vi "ClientSrv Client.vi"() -> ()   [LabVIEW 2012]
doc: "This client VI can connect to a remote server and provides a start menu to open the various user interface windows needed to control and monitor that server. To avoid confusion, no simultaneous connections to multiple servers are allowed. This client and the user interfaces it manages are designed to access a remote server over a TCP/IP network, but are also able to connect to a server running in the same LabVIEW runtime environment. A local connection is convenient for testing during development, and leaves open the option of building a single executable that includes both the client and server. The latter is not advisable since the segregation of the client-side user interfaces from the server not only provides for remote access, but also offloads work and complexity from the server, thereby improving its performance and robustness.\n\nVia the \"server\" menu, a server can be connected to. When a connection to an as yet unkown server is succesfully established, a preset is added that allows a quick reconnection without the need for respecifying the machine name and port number. When disconnecting, the server session is stored. The \"session\" is comprised of the positions, sizes, open/closed state, as well as the persistent controls of the user interface windows. When reconnecting, the previous session is restored.\n\nThe runlevels of the server to which a connection has been established are displayed in a submenu. The attained runlevel is indicated with a checkmark. Using this submenu it is possible to switch the server between runlevels. This operation requires operator access. Note that the runlevels menu does not update while it or some other menu is held open."
uses:
  served/ClientSrv Server Runlevels_srv.ctl
  luaview/served/LuaVIEW Info_srv.ctl
  typedefs/t_ClientSrv Client Main States.ctl
  typedefs/t_ClientSrv Server Runlevels Methods.ctl
  typedefs/t_ClientSrv Access Levels.ctl
  typedefs/t_ClientSrv Client Access State Methods.ctl
  library/typedefs/t_Library Session Methods.ctl
  luaview/typedefs/clusters/LuaVIEW Task Console Ancillary.ctl
  typedefs/t_ClientSrv Connection State Methods.ctl
  subvis/private/glb_ClientSrv Globals.vi
  <vilib>/Platform/browser.llb/Open URL in Default Browser (string).vi
panel:
  in  "local path":path
  in  "editor command":string="notepad \"<file>\""
  out "rebootmode":string
  out "info":T1
  out "runlevels":T2
  out "server":string
  out "remember":bool
  out "observer digest":string
  out "port number":u32
  out "machine name":string
  in  "presets":T3(array[cluster])
  in  "list":i32(listbox)
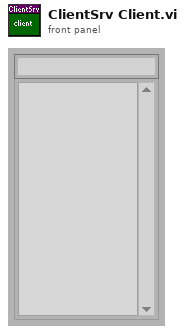
[diagram p1: front panel]
types:
  T1 = typedef "LuaVIEW Info_srv.ctl" = refnum<vi>
  T2 = typedef "ClientSrv Server Runlevels_srv.ctl" = refnum<vi>
  T3 = cluster{"server":string, "machine":string, "port":u32, "digest":string, "remember":bool}[]
  T4 = typedef "t_ClientSrv Client Main States.ctl" = enum16{"empty queue", "poll list selection", "browse editor", "set editor", "no editors?", "<3 editors?", "remote file", "connect", "stop session", "server stop", "server reboot", "disconnect", "open refs", "update presets", "update name", "update ablement", "update sizes", "start session", "run consoles", "initialize", "init title", "init disconnect", "init patience", "init persist", "init paths", "init list", "init sort", "init done", "cleanup", "stop"}
  T5 = typedef "t_ClientSrv Server Runlevels Methods.ctl" = enum16{"get levels", "get modes", "change", "set bootmode"}
  T6 = typedef "t_ClientSrv Access Levels.ctl" = enum16{"observer", "operator", "local"}
  T7 = typedef "t_ClientSrv Client Access State Methods.ctl" = enum16{"ensure", "release"}
  T8 = typedef "LuaVIEW Task Console Ancillary.ctl" = cluster{"open on start":bool, "stop on close":bool, "hide initial":bool, "timeout":u32}
  T9 = typedef "t_Library Session Methods.ctl" = enum16{"run", "get arg", "set arg", "delist", "cleanup?", "start session", "stop session", "list empty?"}
  T10 = typedef "t_ClientSrv Connection State Methods.ctl" = enum16{"connect", "get state", "disconnect"}
  T11 = enum32{"invalid app kind", "Development System", "Run Time System", "Student Edition", "Embedded LabVIEW", "Evaluation", "Custom"}
  T12 = enum32{"existing file", "new file", "new or existing file", "existing dir", "new dir", "new or existing dir", "existing file (use LLBs)", "new file (use LLBs)", "new or existing file (use LLBs)", "new or existing file or directory (use LLBs)"}
  T13 = cluster{"server":string, "machine":string, "port":u32, "digest":string, "remember":bool}
  T14 = typedef "eventvkey.ctl" = enum16{"ASCII", "Enter", "Return", "Shift", "Ctrl", "Alt", "Cmd", "Opt", "Caps", "NumLock", "Clear", "Break", "Up", "Down", "Left", "Right", "Insert", "Delete", "Home", "End", "PageUp", "PageDown", "Escape", "Help", "Pause", "ScrollLock", "F1", "F2", "F3", "F4", "F5", "F6", "F7", "F8", "F9", "F10", "F11", "F12", "F13", "F14", "F15", "F16", "F17", "F18", "F19", "F20", "F21", "F22", "F23", "F24", "Play", "VolumeUp", "VolumeDown", "Mute", "Two Byte Char"}
  T15 = enum32{"Bad", "Idle", "Run top level", "Running"}
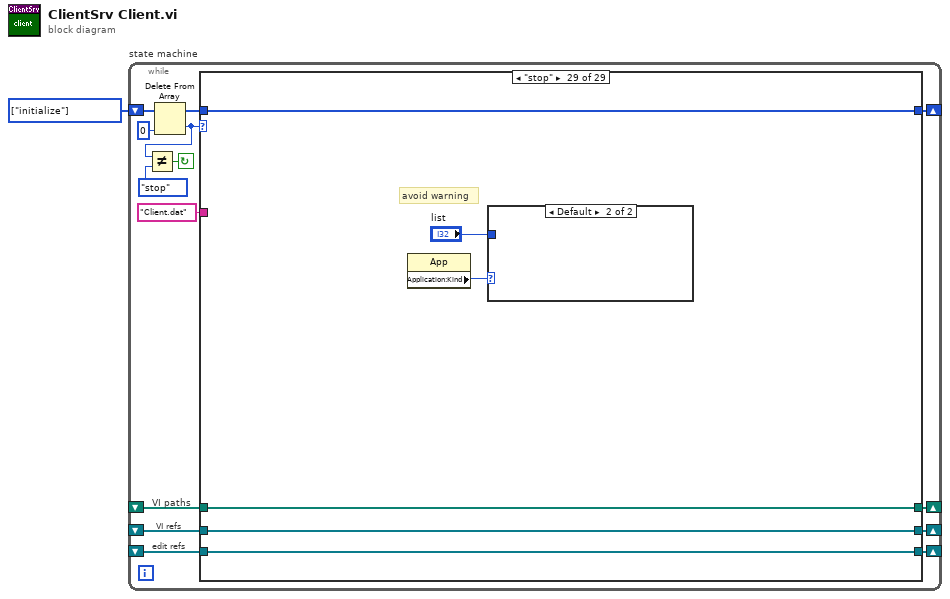
[diagram p0: block diagram]
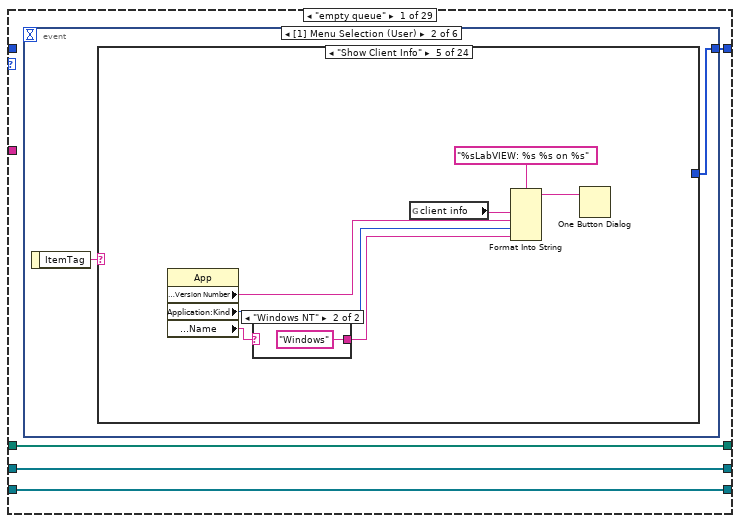
[diagram p2: hidden frame]
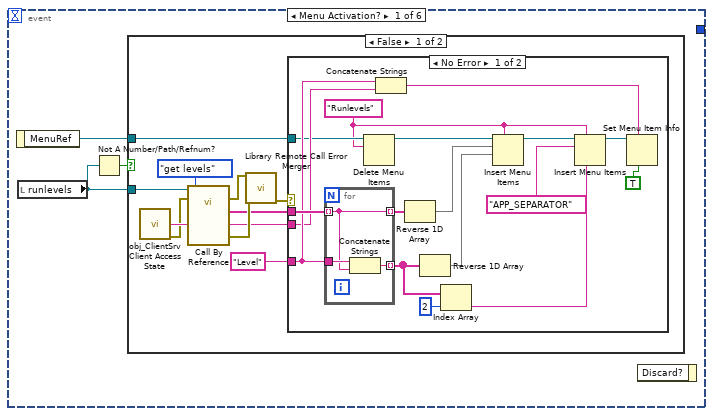
[diagram p3: hidden frame]
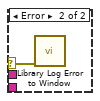
[diagram p4: hidden frame]
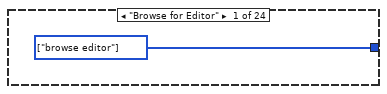
[diagram p6: hidden frame]
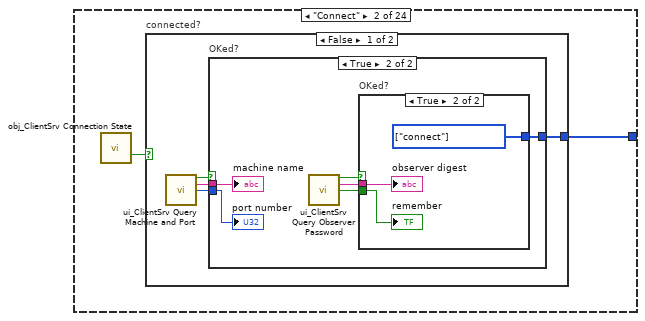
[diagram p7: hidden frame]
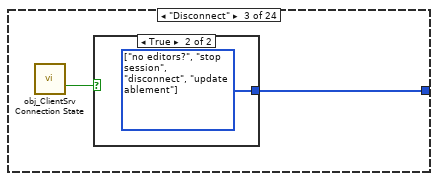
[diagram p11: hidden frame]
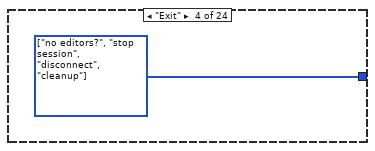
[diagram p13: hidden frame]
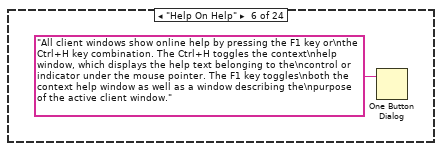
[diagram p15: hidden frame]
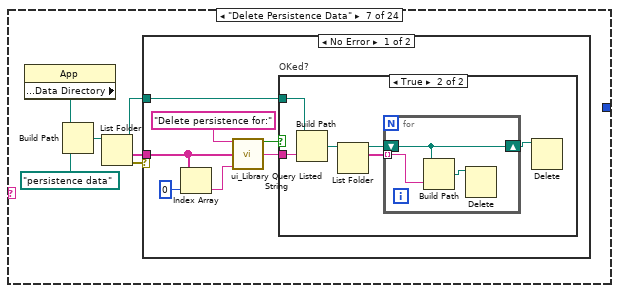
[diagram p16: hidden frame]
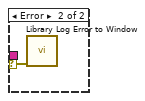
[diagram p18: hidden frame]
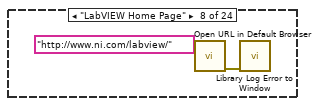
[diagram p19: hidden frame]
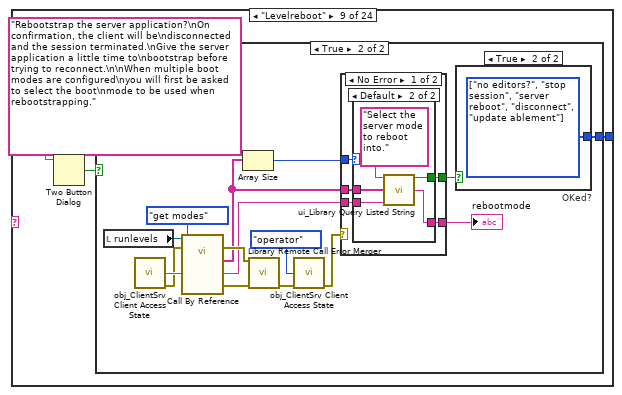
[diagram p20: hidden frame]
diagram:
  w1 = T4[] [enum."initialize"] items=["empty queue", "poll list selection", "browse editor", "set editor", "no editors?", "<3 editors?", "remote file", "connect", "stop session", "server stop", "server reboot", "disconnect", "open refs", "update presets", "update name", "update ablement", "update sizes", "start session", "run consoles", "initialize", "init title", "init disconnect", "init patience", "init persist", "init paths", "init list", "init sort", "init done", "cleanup", "stop"] ("Array Constant")
  n1 = while "state machine" {
    shift-left: w1 -> [w13]
    shift-right: [w15] -> _
    shift-right: [w9] -> _
    shift-left: _ -> [w10]
    shift-right: [w7] -> _
    shift-left: _ -> [w8]
    shift-right: [w3] -> _
    shift-left: _ -> [w2]
    stop <- w14 continue-if-true
    # "edit refs"
    # "VI paths"
    # "VI refs"
    n2 = Delete From Array(array=w13, index=0) -> (deleted portion=w5:T4, array with subset deleted=w12:T4[])  [unwired: 1 in]
    n3 = Not Equal?(x=w5, y=t_ClientSrv_Client_Main_States."stop" ("states")) -> (x != y?=w14:bool)
    n4 = case "Case" shown="\"stop\"" w5 {
      selector: w5 -> [_ _ w318 _ _ _ _ _ _ _ _ _ _ _ _ _ _ _ _ _ _ _ _ _ _ _ _ _ _]
      tunnel: [w19 w309 w322 w345 w369 w408 w424 w430 w455 w460 w479 w508 w570 w604 w647 w668 w673 w689 w693 w722 w727 w736 w740 w753 w771 w852 w865 w882 w892] -> w15
      tunnel: w12 -> [_ w309 w322 w346 w370 w408 _ w430 w455 w460 w479 w508 w570 w604 w647 w668 w673 w689 _ w722 w727 w736 w741 w752 w770 w852 w866 _ w892]
      tunnel: w10 -> [w18 w305 w321 w352 w379 w410 w425 w432 w457 w476 w481 w507 w571 w605 w648 w669 w674 w688 w692 w724 w729 w737 w745 w749 _ w846 w867 w876 w890]
      tunnel: [w18 w305 w321 w352 w379 w410 w425 w432 w457 w476 w481 w507 w571 w605 w648 w669 w674 w688 w692 w724 w729 w737 w745 w749 w766 w846 w867 w875 w890] -> w9
      tunnel: w8 -> [w17 w307 w320 w351 w378 w409 w423 w431 w456 w475 w480 w506 w568 w603 w646 w667 w672 w687 w691 w723 w728 w735 w743 _ w767 w848 w863 w877 w889]
      tunnel: [w17 w306 w320 w351 w378 w409 w423 w431 w456 w475 w480 w506 w568 w603 w646 w667 w672 w687 w691 w723 w728 w735 w743 w750 w767 w847 w863 w878 w889] -> w7
      tunnel: "Client.dat" ("filename (<window title>.dat)") -> [_ _ _ _ _ _ _ _ _ _ _ _ _ _ _ _ _ _ _ _ _ _ w742 _ _ _ _ w871 _]
      tunnel: [w16 w299 w316 w347 w374 w397 w417 w429 w445 w458 w477 w501 w551 w592 w618 w660 w670 w675 w690 w719 w725 w730 w738 w747 w765 w843 w861 w868 w887] -> w3
      tunnel: w2 -> [w16 w299 w316 w350 w377 w396 w417 w429 w445 w458 w477 w501 w551 w592 w618 w660 w670 w675 w690 w719 w725 w730 w738 w747 w765 w843 w861 w868 w887]
      frame "empty queue" {
        n5 = event shown="[1] Menu Selection (User)" {
          selector: _ -> [_ _ _ _ _ _]
          dyn-events: _ -> [_ _ _ _ _ _]
          timeout: _ -> [_ _ _ _ _ _]
          tunnel: [_ w56 w286 _ w297 w298] -> w19
          event Menu Activation? {
            n6 = event-data() -> ("MenuRef"=w20:refnum<k9>)  [unwired: 1 in]
            n7 = local read "runlevels"() -> (w21:T2)
            n8 = Not A Number/Path/Refnum?(number/path/refnum=w21) -> (NaN/Path/Refnum?=w22:bool)
            n9 = case shown="False" w22 {
              tunnel: w21 -> [w33 _]
              tunnel: w20 -> [w23 _]
              frame False {
                n10 = call "obj_ClientSrv Client Access State.vi"() -> ("certificate"=w31:string, "error out"=w30:errorcluster)  [unwired: 14 in]
                n11 = call-by-ref "?"(reference=w33, error in=w30, "method"=t_ClientSrv_Server_Runlevels_Methods."get levels", "certificate"=w31) -> (error out=w29:errorcluster, "names"=w26:string[], "current"=w25:string, 15:"error out"=w28:errorcluster)  [unwired: 11 in, 1 out]
                n12 = call "Library Remote Call Error Merger.vi"("call by reference node error"=w29, "called VI error (no error)"=w28) -> ("error out"=w27:errorcluster)  [unwired: 13 in]
                n13 = case shown="No Error" w27 {
                  selector: w27 -> [_ w54]
                  tunnel: w26 -> [w49 _]
                  tunnel: w25 -> [w47 _]
                  tunnel: "Level" ("menu tag") -> [w48 _]
                  tunnel: w23 -> [w43 _]
                  frame No Error {
                    w41 = "Runlevels" ("menu tag")
                    n14 = for {
                      tunnel: w49 -> [w52] mode=indexing
                      tunnel: [w52] -> w46 mode=indexing
                      tunnel: w48 -> [w53]
                      tunnel: [w51] -> w36 mode=indexing
                      n15 = Concatenate Strings(w53, w52) -> (w51:string)
                    }
                    n16 = Delete Menu Items(8:w41, 9:w43) -> (3:w50:refnum<k9>)  [unwired: 2 in, 1 out]
                    n17 = Concatenate Strings(w48, w47) -> (w45:string)
                    n18 = Reverse 1D Array(array=w46) -> (reversed array=w37:string[])
                    n19 = Reverse 1D Array(array=w36) -> (reversed array=w38:string[])
                    n20 = Index Array(array=w36, index=2) -> (element=w34:string)
                    n21 = Insert Menu Items(5:w41, 7:w38, 8:w37, 9:w50) -> (3:w40:refnum<k9>)  [unwired: 2 in, 2 out]
                    n22 = Insert Menu Items(4:w34, 5:w41, 8:"APP_SEPARATOR" ("after item"), 9:w40) -> (3:w42:refnum<k9>)  [unwired: 2 in, 2 out]
                    n23 = Set Menu Item Info(6:TRUE ("checked"), 7:w45, 11:w42) -> ()  [unwired: 4 in, 2 out]
                  }
                  frame Error {
                    n24 = call "Library Log Error to Window.vi"("error in (no error)"=w54) -> ()  [unwired: 13 in, 2 out]
                  }
                }
              }
              frame True {
              }
            }
            n25 = event-data() -> ()  [unwired: 2 in, 1 out]
          }
          event Menu Selection (User) {
            n26 = event-data() -> ("ItemTag"=w55:string)  [unwired: 1 in]
            n27 = case shown="\"Show Client Info\"" w55 {
              selector: w55 -> [_ _ _ _ _ _ _ _ _ _ _ _ _ _ _ _ _ _ _ _ _ _ _ w201]
              tunnel: [w57 w59 w74 w76 _ _ _ _ w112 w143 _ _ _ _ _ _ _ w174 w175 _ _ _ _ w202] -> w56
              frame "Browse for Editor" {
                w57 = T4[] [enum."browse editor"] items=["empty queue", "poll list selection", "browse editor", "set editor", "no editors?", "<3 editors?", "remote file", "connect", "stop session", "server stop", "server reboot", "disconnect", "open refs", "update presets", "update name", "update ablement", "update sizes", "start session", "run consoles", "initialize", "init title", "init disconnect", "init patience", "init persist", "init paths", "init list", "init sort", "init done", "cleanup", "stop"] ("Array Constant")
              }
              frame "Connect" {
                n28 = call "obj_ClientSrv Connection State.vi"() -> ("connected?"=w58:bool)  [unwired: 8 in, 7 out]
                n29 = case "connected?" shown="False" w58 {
                  tunnel: [w60 _] -> w59
                  frame False {
                    n30 = call "ui_ClientSrv Query Machine and Port.vi"() -> ("OKed?"=w63:bool, "machine name out"=w62:string, "port number out"=w61:u32)  [unwired: 13 in]
                    n31 = case "OKed?" shown="True" w63 {
                      tunnel: w62 -> [_ w68]
                      tunnel: w61 -> [_ w67]
                      tunnel: [_ w69] -> w60
                      frame False {
                      }
                      frame True {
                        n32 = call "ui_ClientSrv Query Observer Password.vi"() -> ("OKed?"=w66:bool, "observer digest"=w65:string, "remember out"=w64:bool)  [unwired: 13 in]
                        n33 = case "OKed?" shown="True" w66 {
                          tunnel: [_ w70] -> w69
                          tunnel: w65 -> [_ w72]
                          tunnel: w64 -> [_ w71]
                          frame False {
                          }
                          frame True {
                            w70 = T4[] [enum."connect"] items=["empty queue", "poll list selection", "browse editor", "set editor", "no editors?", "<3 editors?", "remote file", "connect", "stop session", "server stop", "server reboot", "disconnect", "open refs", "update presets", "update name", "update ablement", "update sizes", "start session", "run consoles", "initialize", "init title", "init disconnect", "init patience", "init persist", "init paths", "init list", "init sort", "init done", "cleanup", "stop"] ("Array Constant")
                            "observer digest" <- w72
                            "remember" <- w71
                          }
                        }
                        "machine name" <- w68
                        "port number" <- w67
                      }
                    }
                  }
                  frame True {
                  }
                }
              }
              frame "Disconnect" {
                n34 = call "obj_ClientSrv Connection State.vi"() -> ("connected?"=w73:bool)  [unwired: 8 in, 7 out]
                n35 = case shown="True" w73 {
                  tunnel: [_ w75] -> w74
                  frame False {
                  }
                  frame True {
                    w75 = T4[] [enum."no editors?", enum."stop session", enum."disconnect", enum."update ablement"] items=["empty queue", "poll list selection", "browse editor", "set editor", "no editors?", "<3 editors?", "remote file", "connect", "stop session", "server stop", "server reboot", "disconnect", "open refs", "update presets", "update name", "update ablement", "update sizes", "start session", "run consoles", "initialize", "init title", "init disconnect", "init patience", "init persist", "init paths", "init list", "init sort", "init done", "cleanup", "stop"] ("Array Constant")
                  }
                }
              }
              frame "Exit" {
                w76 = T4[] [enum."no editors?", enum."stop session", enum."disconnect", enum."cleanup"] items=["empty queue", "poll list selection", "browse editor", "set editor", "no editors?", "<3 editors?", "remote file", "connect", "stop session", "server stop", "server reboot", "disconnect", "open refs", "update presets", "update name", "update ablement", "update sizes", "start session", "run consoles", "initialize", "init title", "init disconnect", "init patience", "init persist", "init paths", "init list", "init sort", "init done", "cleanup", "stop"] ("Array Constant")
              }
              frame "Show Client Info" {
                n36 = property class="App"() -> ("Application:Version Number"=w82:string, "Application:Kind"=w81:T11, "Operating System:Name"=w80:string)  [unwired: 2 in, 2 out]
                n37 = case shown="\"Windows NT\"" w80 {
                  selector: w80 -> [w84 _]
                  tunnel: [w84 "Windows"] -> w79
                  frame Default {
                  }
                  frame "Windows NT" {
                  }
                }
                n38 = global read "glb_ClientSrv Globals.vi" "client info"() -> (w77:string)
                n39 = Format Into String(format string="%sLabVIEW: %s %s on %s", w77, w82, w81, w79) -> (resulting string=w78:string)  [unwired: 2 in, 1 out]
                n40 = One Button Dialog(message=w78) -> ()  [unwired: 1 in, 1 out]
              }
              frame "Help On Help" {
                n41 = One Button Dialog(message="All client windows show online help by pressing the F1 key or\nthe Ctrl+H key combination. The Ctrl+H toggles the context\nhelp window, which displays the help text belonging to the\ncontrol or indicator under the mouse pointer. The F1 key toggles\nboth the context help window as well as a window describing the\npurpose of the active client window.") -> ()  [unwired: 1 in, 1 out]
              }
              frame "Delete Persistence Data" {
                n42 = property class="App"() -> ("Application:Default:Data Directory"=w91:path)  [unwired: 2 in, 2 out]
                n43 = Build Path(base path=w91, name or relative path=path "persistence data" ("path in")) -> (appended path=w90:path)
                n44 = List Folder(path=w90) -> (path out=w87:path, folder names=w88:string[], error out=w89:errorcluster)  [unwired: 3 in, 1 out]
                n45 = case shown="No Error" w89 {
                  selector: w89 -> [_ w109]
                  tunnel: w88 -> [w97 _]
                  tunnel: w87 -> [w95 _]
                  frame No Error {
                    n46 = Index Array(array=w97, index=0) -> (element=w98:string)
                    n47 = call "ui_Library Query Listed String.vi"("prompt"="Delete persistence for:", "list of strings"=w97, "default (persist)"=w98) -> ("OKed?"=w93:bool, "selected string"=w94:string)  [unwired: 11 in]
                    n48 = case "OKed?" shown="True" w93 {
                      tunnel: w95 -> [_ w105]
                      tunnel: w94 -> [_ w104]
                      frame False {
                      }
                      frame True {
                        n49 = Build Path(base path=w105, name or relative path=w104) -> (appended path=w103:path)
                        n50 = List Folder(path=w103) -> (path out=w102:path, filenames=w100:string[])  [unwired: 3 in, 2 out]
                        n51 = for {
                          shift-right: [w107] -> w101
                          shift-left: w102 -> [w107]
                          tunnel: w100 -> [w108] mode=indexing
                          n52 = Build Path(base path=w107, name or relative path=w108) -> (appended path=w106:path)
                          n53 = Delete(path (use dialog)=w106) -> ()  [unwired: 4 in, 3 out]
                        }
                        n54 = Delete(path (use dialog)=w101) -> ()  [unwired: 4 in, 3 out]
                      }
                    }
                  }
                  frame Error {
                    n55 = call "Library Log Error to Window.vi"("error in (no error)"=w109) -> ()  [unwired: 13 in, 2 out]
                  }
                }
              }
              frame "LabVIEW Home Page" {
                n56 = call-poly <vilib>:"Open URL in Default Browser.vi"("URL"="http://www.ni.com/labview/") -> ("error out"=w111:errorcluster)  [unwired: 5 in, 1 out]
                n57 = call "Library Log Error to Window.vi"("error in (no error)"=w111) -> ()  [unwired: 13 in, 2 out]
              }
              frame "Levelreboot" {
                n58 = Two Button Dialog(message="Rebootstrap the server application?\nOn confirmation, the client will be\ndisconnected and the session terminated.\nGive the server application a little time to\nbootstrap before trying to reconnect.\n\nWhen multiple boot modes are configured\nyou will first be asked to select the boot\nmode to be used when rebootstrapping." ("format string")) -> (T button?=w113:bool)  [unwired: 2 in]
                n59 = case shown="True" w113 {
                  tunnel: [_ w129] -> w112
                  frame False {
                  }
                  frame True {
                    n60 = local read "runlevels"() -> (w123:T2)
                    n61 = call "obj_ClientSrv Client Access State.vi"() -> ("certificate"=w127:string, "error out"=w126:errorcluster)  [unwired: 14 in]
                    n62 = call-by-ref "?"(reference=w123, error in=w126, "method"=t_ClientSrv_Server_Runlevels_Methods."get modes", "certificate"=w127) -> (error out=w125:errorcluster, "names"=w121:string[], "current"=w122:string, 15:"error out"=w124:errorcluster)  [unwired: 11 in, 1 out]
                    n63 = Array Size(array=w121) -> (size(s)=w120:i32)
                    n64 = call "Library Remote Call Error Merger.vi"("call by reference node error"=w125, "called VI error (no error)"=w124) -> ("error out"=w117:errorcluster)  [unwired: 13 in]
                    n65 = call "obj_ClientSrv Client Access State.vi"("access level (observer)"=t_ClientSrv_Access_Levels."operator" ("access level in"), "error in (no error)"=w117) -> ("error out"=w116:errorcluster)  [unwired: 12 in, 1 out]
                    n66 = case shown="No Error" w116 {
                      selector: w116 -> [_ w141]
                      tunnel: w122 -> [w134 _]
                      tunnel: w121 -> [w133 _]
                      tunnel: w120 -> [w132 _]
                      tunnel: [w131 _] -> w119
                      tunnel: [w130 _] -> w118
                      frame No Error {
                        n67 = case shown="Default" w132 {
                          tunnel: w133 -> [_ w140]
                          tunnel: w134 -> [_ w139]
                          tunnel: [TRUE w137] -> w130
                          tunnel: [_ w138] -> w131
                          frame 0 {
                          }
                          frame Default {
                            n68 = call "ui_Library Query Listed String.vi"("prompt"="Select the server mode to reboot into.", "list of strings"=w140, "default (persist)"=w139) -> ("OKed?"=w137:bool, "selected string"=w138:string)  [unwired: 11 in]
                          }
                        }
                      }
                      frame Error {
                        n69 = call "Library Log Error to Window.vi"("error in (no error)"=w141) -> ()  [unwired: 13 in, 2 out]
                      }
                    }
                    "rebootmode" <- w119
                    n70 = case "OKed?" shown="True" w118 {
                      tunnel: [_ w142] -> w129
                      frame False {
                      }
                      frame True {
                        w142 = T4[] [enum."no editors?", enum."stop session", enum."server reboot", enum."disconnect", enum."update ablement"] items=["empty queue", "poll list selection", "browse editor", "set editor", "no editors?", "<3 editors?", "remote file", "connect", "stop session", "server stop", "server reboot", "disconnect", "open refs", "update presets", "update name", "update ablement", "update sizes", "start session", "run consoles", "initialize", "init title", "init disconnect", "init patience", "init persist", "init paths", "init list", "init sort", "init done", "cleanup", "stop"] ("Array Constant")
                      }
                    }
                  }
                }
              }
              frame "Levelstop" {
                n71 = Two Button Dialog(message="Stop the server application?\nThe client will be disconnected\nand the session terminated." ("format string")) -> (T button?=w144:bool)  [unwired: 2 in]
                n72 = case shown="True" w144 {
                  tunnel: [_ w148] -> w143
                  frame False {
                  }
                  frame True {
                    n73 = call "obj_ClientSrv Client Access State.vi"("access level (observer)"=t_ClientSrv_Access_Levels."operator" ("access level in")) -> ("error out"=w146:errorcluster)  [unwired: 13 in, 1 out]
                    n74 = case shown="No Error" w146 {
                      tunnel: [w149 _] -> w148
                      frame No Error {
                        w149 = T4[] [enum."no editors?", enum."stop session", enum."server stop", enum."disconnect", enum."update ablement"] items=["empty queue", "poll list selection", "browse editor", "set editor", "no editors?", "<3 editors?", "remote file", "connect", "stop session", "server stop", "server reboot", "disconnect", "open refs", "update presets", "update name", "update ablement", "update sizes", "start session", "run consoles", "initialize", "init title", "init disconnect", "init patience", "init persist", "init paths", "init list", "init sort", "init done", "cleanup", "stop"] ("Array Constant")
                      }
                      frame Error {
                      }
                    }
                  }
                }
              }
              frame "Local File" {
                (unwired) T12."existing file" ("select mode (2)")
                n75 = File Dialog(5:"Select" ("button label"), 7:"Select a file to edit:" ("prompt"), 11:"local path") -> (1:w152:bool, 3:w151:path)  [unwired: 4 in, 2 out]
                n76 = case "cancelled?" shown="False" w152 {
                  tunnel: w151 -> [w160 _]
                  frame False {
                    n77 = Path To String(path=w160) -> (string=w157:string)
                    n78 = Strip Path(path=w160) -> (stripped path=w159:path)  [unwired: 1 out]
                    n79 = Search and Replace String(input string="editor command", search string="<file>", replace string=w157) -> (result string=w158:string)  [unwired: 5 in, 3 out]
                    n80 = local write "local path"(w159) -> ()
                    n81 = call <vilib>:"System Exec.vi"("wait until completion? (T)"=FALSE, "command line"=w158) -> ("error out"=w161:errorcluster)  [unwired: 6 in, 3 out]
                    n82 = call "Library Log Error to Window.vi"("error in (no error)"=w161) -> ()  [unwired: 13 in, 2 out]
                  }
                  frame True {
                  }
                }
              }
              frame "Lua Book" {
                n83 = call-poly <vilib>:"Open URL in Default Browser.vi"("URL"="http://www.lua.org/pil/") -> ("error out"=w164:errorcluster)  [unwired: 5 in, 1 out]
                n84 = call "Library Log Error to Window.vi"("error in (no error)"=w164) -> ()  [unwired: 13 in, 2 out]
              }
              frame "Lua Home Page" {
                n85 = call-poly <vilib>:"Open URL in Default Browser.vi"("URL"="http://www.lua.org/") -> ("error out"=w166:errorcluster)  [unwired: 5 in, 1 out]
                n86 = call "Library Log Error to Window.vi"("error in (no error)"=w166) -> ()  [unwired: 13 in, 2 out]
              }
              frame "Lua Reference Manual" {
                n87 = call-poly <vilib>:"Open URL in Default Browser.vi"("URL"="http://www.lua.org/manual/5.0/") -> ("error out"=w168:errorcluster)  [unwired: 5 in, 1 out]
                n88 = call "Library Log Error to Window.vi"("error in (no error)"=w168) -> ()  [unwired: 13 in, 2 out]
              }
              frame "LuaVIEW Home Page" {
                n89 = call-poly <vilib>:"Open URL in Default Browser.vi"("URL"="http://www.citengineering.com/luaview/") -> ("error out"=w170:errorcluster)  [unwired: 5 in, 1 out]
                n90 = call "Library Log Error to Window.vi"("error in (no error)"=w170) -> ()  [unwired: 13 in, 2 out]
              }
              frame "LuaVIEW Manual" {
                n91 = call-poly <vilib>:"Open URL in Default Browser.vi"("URL"="http://www.citengineering.com/LuaVIEW/manual.html") -> ("error out"=w172:errorcluster)  [unwired: 5 in, 1 out]
                n92 = call "Library Log Error to Window.vi"("error in (no error)"=w172) -> ()  [unwired: 13 in, 2 out]
              }
              frame "Release Access" {
                n93 = call "obj_ClientSrv Client Access State.vi"("method (ensure)"=t_ClientSrv_Client_Access_State_Methods."release") -> ()  [unwired: 13 in, 2 out]
              }
              frame "Remote File" {
                w174 = T4[] [enum."<3 editors?", enum."remote file"] items=["empty queue", "poll list selection", "browse editor", "set editor", "no editors?", "<3 editors?", "remote file", "connect", "stop session", "server stop", "server reboot", "disconnect", "open refs", "update presets", "update name", "update ablement", "update sizes", "start session", "run consoles", "initialize", "init title", "init disconnect", "init patience", "init persist", "init paths", "init list", "init sort", "init done", "cleanup", "stop"] ("Array Constant")
              }
              frame "Set Editor Command" {
                w175 = T4[] [enum."set editor"] items=["empty queue", "poll list selection", "browse editor", "set editor", "no editors?", "<3 editors?", "remote file", "connect", "stop session", "server stop", "server reboot", "disconnect", "open refs", "update presets", "update name", "update ablement", "update sizes", "start session", "run consoles", "initialize", "init title", "init disconnect", "init patience", "init persist", "init paths", "init list", "init sort", "init done", "cleanup", "stop"] ("Array Constant")
              }
              frame "Show Client Errors" {
                n94 = call "ui_Library Error Log Window.vi"() -> ()  [unwired: 2 in]
              }
              frame "Show Server Errors" {
                n95 = call "Library Resolve VI Path.vi"("VI name"="ui_LuaVIEW Task Console.vit", "sub path of toolkit (none)"=path "dynamic" ("subdirectory of tree (none)")) -> ("VI path"=w179:path)  [unwired: 13 in]
                n96 = Flatten To String(anything=T8 {"open on start"=TRUE, "stop on close"=FALSE, "hide initial"=FALSE, "timeout"=0} ("task console ancillary")) -> (data string=w177:string)  [unwired: 3 in, 2 out]
                n97 = call "obj_Library Session.vi"("method"=t_Library_Session_Methods."run", "path"=w179, "argument in (none)"="errors", "ancillary in (none)"=w177) -> ("error out"=w180:errorcluster)  [unwired: 8 in, 3 out]
                n98 = call "Library Log Error to Window.vi"("error in (no error)"=w180) -> ()  [unwired: 13 in, 2 out]
              }
              frame "Show Server Info" {
                n99 = call "obj_ClientSrv Client Access State.vi"() -> ("certificate"=w189:string, "error out"=w188:errorcluster)  [unwired: 14 in]
                n100 = local read "info"() -> (w190:T1)
                n101 = call-by-ref "?"(reference=w190, error in=w188, "certificate"=w189) -> (error out=w186:errorcluster, "info"=w184:string, 15:"error out"=w187:errorcluster)  [unwired: 13 in, 1 out]
                n102 = call "Library Remote Call Error Merger.vi"("call by reference node error"=w186, "called VI error (no error)"=w187) -> ("error out"=w185:errorcluster)  [unwired: 13 in]
                n103 = case shown="No Error" w185 {
                  selector: w185 -> [_ w192]
                  tunnel: w184 -> [w191 _]
                  frame No Error {
                    n104 = One Button Dialog(message=w191) -> ()  [unwired: 1 in, 1 out]
                  }
                  frame Error {
                    n105 = call "Library Log Error to Window.vi"("error in (no error)"=w192) -> ()  [unwired: 13 in, 2 out]
                  }
                }
              }
              frame "Show Server Warnings" {
                n106 = call "Library Resolve VI Path.vi"("VI name"="ui_LuaVIEW Task Console.vit", "sub path of toolkit (none)"=path "dynamic" ("subdirectory of tree (none)")) -> ("VI path"=w196:path)  [unwired: 13 in]
                n107 = Flatten To String(anything=T8 {"open on start"=TRUE, "stop on close"=FALSE, "hide initial"=FALSE, "timeout"=0} ("task console ancillary")) -> (data string=w193:string)  [unwired: 3 in, 2 out]
                n108 = call "obj_Library Session.vi"("method"=t_Library_Session_Methods."run", "path"=w196, "argument in (none)"="warnings", "ancillary in (none)"=w193) -> ("error out"=w197:errorcluster)  [unwired: 8 in, 3 out]
                n109 = call "Library Log Error to Window.vi"("error in (no error)"=w197) -> ()  [unwired: 13 in, 2 out]
              }
              frame Default {
                n110 = Match Pattern(string=w201, regular expression="^Preset") -> (after substring=w203:string, offset past match=w205:i32)  [unwired: 1 in, 2 out]
                n111 = Greater Or Equal To 0?(x=w205) -> (x >= 0?=w204:bool)
                n112 = case shown="True" w204 {
                  tunnel: w203 -> [_ w249]
                  tunnel: [w207 w250] -> w202
                  tunnel: w201 -> [w209 _]
                  frame False {
                    n113 = Match Pattern(string=w209, regular expression="^Remove") -> (after substring=w208:string, offset past match=w212:i32)  [unwired: 1 in, 2 out]
                    n114 = Greater Or Equal To 0?(x=w212) -> (x >= 0?=w210:bool)
                    n115 = case shown="False" w210 {
                      tunnel: w209 -> [w215 _]
                      tunnel: w208 -> [_ w242]
                      tunnel: [_ w239] -> w207
                      frame False {
                        n116 = Match Pattern(string=w215, regular expression="^Level") -> (after substring=w213:string, offset past match=w216:i32)  [unwired: 1 in, 2 out]
                        n117 = Greater Or Equal To 0?(x=w216) -> (x >= 0?=w214:bool)
                        n118 = case shown="True" w214 {
                          tunnel: w215 -> [w218 _]
                          tunnel: w213 -> [_ w222]
                          frame False {
                            n119 = Format Into String(format string="Unhandled menu tag \"%s\"", w218) -> (resulting string=w219:string)  [unwired: 2 in, 1 out]
                            n120 = One Button Dialog(message=w219) -> ()  [unwired: 1 in, 1 out]
                          }
                          frame True {
                            n121 = Format Into String(format string="Switch server to runlevel \"%s\"?", w222) -> (resulting string=w223:string)  [unwired: 2 in, 1 out]
                            n122 = Two Button Dialog(message=w223) -> (T button?=w221:bool)  [unwired: 2 in]
                            n123 = case shown="True" w221 {
                              tunnel: w222 -> [_ w227]
                              frame False {
                              }
                              frame True {
                                n124 = local read "runlevels"() -> (w226:T2)
                                n125 = call "obj_ClientSrv Client Access State.vi"("access level (observer)"=t_ClientSrv_Access_Levels."operator") -> ("certificate"=w232:string, "error out"=w231:errorcluster)  [unwired: 13 in]
                                n126 = call-by-ref "?"(reference=w226, error in=w231, "method"=t_ClientSrv_Server_Runlevels_Methods."change", "certificate"=w232, "runlevel/bootmode"=w227) -> (error out=w230:errorcluster, 15:"error out"=w229:errorcluster)  [unwired: 10 in, 3 out]
                                n127 = call "Library Remote Call Error Merger.vi"("call by reference node error"=w230, "called VI error (no error)"=w229) -> ("error out"=w225:errorcluster)  [unwired: 13 in]
                                n128 = call "Library Log Error to Window.vi"("error in (no error)"=w225) -> ()  [unwired: 13 in, 2 out]
                              }
                            }
                          }
                        }
                      }
                      frame True {
                        n129 = Decimal String To Number(string=w242) -> (number=w240:i32)  [unwired: 2 in, 1 out]
                        n130 = local read "presets"() -> (w241:T3)
                        n131 = Index Array(array=w241, index=w240) -> (element=w238:T13)
                        n132 = Unbundle By Name(w238) -> ("server"=w237:string)
                        n133 = Format Into String(format string="Remove preset for server \"%s\"?", w237) -> (resulting string=w235:string)  [unwired: 2 in, 1 out]
                        n134 = Two Button Dialog(message=w235) -> (T button?=w234:bool)  [unwired: 2 in]
                        n135 = case shown="True" w234 {
                          tunnel: w241 -> [_ w245]
                          tunnel: w240 -> [_ w244]
                          tunnel: [_ w243] -> w239
                          frame False {
                          }
                          frame True {
                            w243 = T4[] [enum."update ablement"] items=["empty queue", "poll list selection", "browse editor", "set editor", "no editors?", "<3 editors?", "remote file", "connect", "stop session", "server stop", "server reboot", "disconnect", "open refs", "update presets", "update name", "update ablement", "update sizes", "start session", "run consoles", "initialize", "init title", "init disconnect", "init patience", "init persist", "init paths", "init list", "init sort", "init done", "cleanup", "stop"] ("Array Constant")
                            n136 = Delete From Array(array=w245, index=w244) -> (array with subset deleted=w246:T3)  [unwired: 1 in, 1 out]
                            n137 = local write "presets"(w246) -> ()
                          }
                        }
                      }
                    }
                  }
                  frame True {
                    n138 = local read "presets"() -> (w259:T3)
                    n139 = Decimal String To Number(string=w249) -> (number=w248:i32)  [unwired: 2 in, 1 out]
                    n140 = Index Array(array=w259, index=w248) -> (element=w258:T13)
                    n141 = Unbundle By Name(w258) -> ("machine"=w257:string, "port"=w256:u32, "digest"=w254:string, "remember"=w255:bool, "server"=w247:string)
                    n142 = case shown="False" w255 {
                      selector: w255 -> [_ w283]
                      tunnel: [w281 w284] -> w252
                      tunnel: w254 -> [_ w284]
                      tunnel: [w280 w283] -> w251
                      tunnel: [w279 TRUE ("OKed?")] -> w253
                      frame False {
                        n143 = call "ui_ClientSrv Query Observer Password.vi"() -> ("OKed?"=w279:bool, "observer digest"=w281:string, "remember out"=w280:bool)  [unwired: 13 in]
                      }
                      frame True {
                      }
                    }
                    n144 = case shown="True" w253 {
                      tunnel: [w260 w268] -> w250
                      tunnel: w257 -> [_ w263]
                      tunnel: w256 -> [_ w264]
                      tunnel: w252 -> [_ w262]
                      tunnel: w251 -> [_ w265]
                      tunnel: w247 -> [_ w261]
                      frame False {
                        w260 = T4[] [enum."update ablement"] items=["empty queue", "poll list selection", "browse editor", "set editor", "no editors?", "<3 editors?", "remote file", "connect", "stop session", "server stop", "server reboot", "disconnect", "open refs", "update presets", "update name", "update ablement", "update sizes", "start session", "run consoles", "initialize", "init title", "init disconnect", "init patience", "init persist", "init paths", "init list", "init sort", "init done", "cleanup", "stop"] ("Array Constant")
                      }
                      frame True {
                        n145 = call "obj_ClientSrv Connection State.vi"("method (get state)"=t_ClientSrv_Connection_State_Methods."connect" ("method"), "machine{connect}/VI{get state} name (local/no path resolution)"=w263, "port number in (3363)"=w264, "observer digest"=w262) -> ("error out"=w266:errorcluster)  [unwired: 4 in, 7 out]
                        n146 = case shown="No Error" w266 {
                          selector: w266 -> [_ w278]
                          tunnel: [w273 w277] -> w268
                          tunnel: w263 -> [w272 _]
                          tunnel: w264 -> [w271 _]
                          tunnel: w265 -> [w270 _]
                          tunnel: w262 -> [w269 _]
                          tunnel: w261 -> [_ w275]
                          frame No Error {
                            w273 = T4[] [enum."open refs", enum."update presets", enum."update name", enum."update ablement", enum."start session", enum."run consoles"] items=["empty queue", "poll list selection", "browse editor", "set editor", "no editors?", "<3 editors?", "remote file", "connect", "stop session", "server stop", "server reboot", "disconnect", "open refs", "update presets", "update name", "update ablement", "update sizes", "start session", "run consoles", "initialize", "init title", "init disconnect", "init patience", "init persist", "init paths", "init list", "init sort", "init done", "cleanup", "stop"] ("Array Constant")
                            n147 = local write "machine name"(w272) -> ()
                            n148 = local write "port number"(w271) -> ()
                            n149 = local write "observer digest"(w269) -> ()
                            n150 = local write "remember"(w270) -> ()
                          }
                          frame Error {
                            w277 = T4[] [enum."update ablement"] items=["empty queue", "poll list selection", "browse editor", "set editor", "no editors?", "<3 editors?", "remote file", "connect", "stop session", "server stop", "server reboot", "disconnect", "open refs", "update presets", "update name", "update ablement", "update sizes", "start session", "run consoles", "initialize", "init title", "init disconnect", "init patience", "init persist", "init paths", "init list", "init sort", "init done", "cleanup", "stop"] ("Array Constant")
                            n151 = call "Library Log Error to Window.vi"("error in (no error)"=w278) -> ()  [unwired: 13 in, 2 out]
                            n152 = Format Into String(format string="Could not connect to preset server \"%s\".\nLikely, there is trouble with the network connection\nor the server has been shut down.\nHowever it might be that the server was moved to\na different machine or port, in which case \"Connect\"\nshould be used and the new machine/port entered.\nIf the server has ceased to exist altogether,\nuse \"Remove Preset\"." ("message"), w275) -> (resulting string=w274:string)  [unwired: 2 in, 1 out]
                            n153 = One Button Dialog(message=w274) -> ()  [unwired: 1 in, 1 out]
                          }
                        }
                      }
                    }
                  }
                }
              }
            }
          }
          event Key Down? {
            n154 = event-data() -> ("VKey"=w285:T14)  [unwired: 1 in]
            n155 = call <vilib>:"compatReturnToEnter.vi"("VKey"=w285) -> ("VKey"=w288:T14)
            n156 = case shown="\"F1\"" w288 {
              tunnel: [TRUE ("Discard?") _ _ _] -> w287
              tunnel: [_ w291 _ _] -> w286
              frame "F1" {
                n157 = call "Library Show Help.vi"() -> ()  [unwired: 1 in]
              }
              frame "Enter" {
                w291 = T4[] [enum."poll list selection"] items=["empty queue", "poll list selection", "browse editor", "set editor", "no editors?", "<3 editors?", "remote file", "connect", "stop session", "server stop", "server reboot", "disconnect", "open refs", "update presets", "update name", "update ablement", "update sizes", "start session", "run consoles", "initialize", "init title", "init disconnect", "init patience", "init persist", "init paths", "init list", "init sort", "init done", "cleanup", "stop"] ("Array Constant")
                n158 = property on="list" class="LstBox (strict)"("Key Focus"=TRUE) -> ()  [unwired: 2 in, 2 out]
              }
              frame Default {
              }
              frame "Up", "Down" {
                n159 = property on="list" class="LstBox (strict)"("Key Focus"=TRUE) -> ()  [unwired: 2 in, 2 out]
              }
            }
            n160 = event-data("Discard?"=w287) -> ()  [unwired: 1 in, 1 out]
          }
          event event type 5.0.x8000000b {
            n161 = event-data() -> ("VKey"=w293:T14)  [unwired: 1 in]
            n162 = call <vilib>:"compatReturnToEnter.vi"("VKey"=w293) -> ("VKey"=w295:T14)
            n163 = case shown="\"F1\"" w295 {
              tunnel: [_ TRUE] -> w294
              frame Default {
              }
              frame "F1" {
              }
            }
            n164 = event-data("Discard?"=w294) -> ()  [unwired: 1 in, 1 out]
          }
          event Mouse Up {
            w297 = T4[] [enum."poll list selection"] items=["empty queue", "poll list selection", "browse editor", "set editor", "no editors?", "<3 editors?", "remote file", "connect", "stop session", "server stop", "server reboot", "disconnect", "open refs", "update presets", "update name", "update ablement", "update sizes", "start session", "run consoles", "initialize", "init title", "init disconnect", "init patience", "init persist", "init paths", "init list", "init sort", "init done", "cleanup", "stop"] ("Array Constant")
            # "Cheaply monitor list selection\nthrough double clicks.\nA double click is not registered\nuntil the mouse is released a\nsecond time."
            n165 = event-data() -> ()  [unwired: 1 in, 1 out]
          }
          event Panel Resize {
            w298 = T4[] [enum."update sizes"] items=["empty queue", "poll list selection", "browse editor", "set editor", "no editors?", "<3 editors?", "remote file", "connect", "stop session", "server stop", "server reboot", "disconnect", "open refs", "update presets", "update name", "update ablement", "update sizes", "start session", "run consoles", "initialize", "init title", "init disconnect", "init patience", "init persist", "init paths", "init list", "init sort", "init done", "cleanup", "stop"] ("Array Constant")
            n166 = event-data() -> ()  [unwired: 1 in, 1 out]
          }
        }
      }
      frame "poll list selection" {
        w303 = u8 0 items=["enabled", "disabled", "grayed"] ("disabled state")
        n167 = property on="list" class="LstBox (strict)"() -> ("Double-Click"=w308:i32, "Disabled"=w302:u8)  [unwired: 2 in, 2 out]
        n168 = Equal?(x=w302, y=w303) -> (x = y?=w301:bool)
        n169 = Greater Or Equal To 0?(x=w308) -> (x >= 0?=w304:bool)
        n170 = And(x=w304, y=w301) -> (x .and. y?=w300:bool)
        n171 = case shown="True" w300 {
          tunnel: w308 -> [_ w315]
          tunnel: w307 -> [w310 w311]
          tunnel: [w310 w311] -> w306
          frame False {
          }
          frame True {
            n172 = Index Array(array=w311, index=w315) -> (element=w314:path)
            n173 = call "obj_Library Session.vi"("method"=t_Library_Session_Methods."run", "path"=w314) -> ("error out"=w312:errorcluster)  [unwired: 10 in, 3 out]
            n174 = call "Library Log Error to Window.vi"("error in (no error)"=w312) -> ()  [unwired: 13 in, 2 out]
          }
        }
      }
      frame "browse editor", "set editor" {
        n175 = case shown="\"browse editor\"" w318 {
          tunnel: [TRUE ("cancelled") _ w331] -> w319
          tunnel: [_ w324 w326] -> w317
          frame Default {
          }
          frame "set editor" {
            n176 = local read "editor command"() -> (w324:string)
          }
          frame "browse editor" {
            (unwired) T12."existing file" ("select mode (2)")
            n177 = File Dialog(5:"Select" ("button label"), 7:"Select an editor executable:" ("prompt")) -> (1:w331:bool, 3:w327:path)  [unwired: 5 in, 2 out]
            n178 = Path To String(path=w327) -> (string=w330:string)
            n179 = Concatenate Strings("\"" ("string"), w330, "\" \"<file>\"" ("string")) -> (w326:string)
          }
        }
        n180 = case "cancelled?" shown="False" w319 {
          tunnel: w317 -> [w333 _]
          frame False {
            n181 = call "ui_Library Query String.vi"("prompt"="Set Editor Command", "string in (\"\")"=w333) -> ("OKed?"=w335:bool, "string out"=w334:string)  [unwired: 12 in]
            n182 = case "OKed?" shown="True" w335 {
              tunnel: w334 -> [_ w337]
              frame False {
              }
              frame True {
                n183 = Search/Split String(string=w337, search string/char (-)="<file>") -> (offset of match=w339:i32)  [unwired: 1 in, 2 out]
                n184 = Greater Or Equal To 0?(x=w339) -> (x >= 0?=w338:bool)
                n185 = case shown="False" w338 {
                  tunnel: w337 -> [_ w342]
                  frame False {
                    n186 = One Button Dialog(message="Invalid editor command.\nThe command line must contain the substring <file>\nwhich, before execution, is substituted with the\npath to the file to be edited. Place double quotes\nbefore and after this substring to allow for the\npresence of spaces in the path.") -> ()  [unwired: 1 in, 1 out]
                  }
                  frame True {
                    n187 = local write "editor command"(w342) -> ()
                  }
                }
              }
            }
          }
          frame True {
          }
        }
      }
      frame "no editors?" {
        n188 = for {
          tunnel: w350 -> [w361] mode=indexing
          shift-right: [w358] -> w344
          shift-left: 0 -> [w359]
          shift-right: [w355] -> w347
          shift-left: refnum<vi>[] [] -> [w356]
          n189 = property class="VI"(reference=w361) -> (reference out=w357:refnum<vi>, "Execution:State"=w360:T15)  [unwired: 1 in, 1 out]
          n190 = case shown="\"Run top level\"" w360 {
            tunnel: w359 -> [w366 w368]
            tunnel: [w365 w368] -> w358
            tunnel: w357 -> [w362 _]
            tunnel: w356 -> [w364 w367]
            tunnel: [w363 w367] -> w355
            frame "Run top level" {
              n191 = Increment(x=w366) -> (x+1=w365:i32)
              n192 = Build Array (concatenate)(w364, w362) -> (w363:refnum<vi>[])
            }
            frame Default {
            }
          }
        }
        n193 = Greater Than 0?(x=w344) -> (x > 0?=w343:bool)
        n194 = case shown="True" w343 {
          tunnel: w346 -> [w353 _]
          tunnel: [w353 _] -> w345
          frame False {
          }
          frame True {
            n195 = One Button Dialog(message="Operation cancelled: there are still\nremote files being edited. To be able\nto disconnect from the server, all\neditors must first be closed.") -> ()  [unwired: 1 in, 1 out]
          }
        }
      }
      frame "<3 editors?" {
        # "Since \"System Exec\" is used which calls into C to spawn the editor, each open editor occupies a thread. Though the \"Other 2\"\nexecution system is used, we do not want to use up all threads in\nthis execution system since there is a small chance that it is\nused elsewehere. Thus we allow up to three simultaneously\nactive editors, thereby leaving at least one \"Other 2\" thread in\ncase of the normal four thread per execution system configuration."
        n196 = for {
          tunnel: w377 -> [w388] mode=indexing
          shift-right: [w385] -> w373
          shift-left: 0 -> [w386]
          shift-right: [w382] -> w374
          shift-left: refnum<vi>[] [] -> [w383]
          n197 = property class="VI"(reference=w388) -> (reference out=w384:refnum<vi>, "Execution:State"=w387:T15)  [unwired: 1 in, 1 out]
          n198 = case shown="\"Run top level\"" w387 {
            tunnel: w386 -> [w393 w395]
            tunnel: [w392 w395] -> w385
            tunnel: w384 -> [w389 _]
            tunnel: w383 -> [w391 w394]
            tunnel: [w390 w394] -> w382
            frame "Run top level" {
              n199 = Increment(x=w393) -> (x+1=w392:i32)
              n200 = Build Array (concatenate)(w391, w389) -> (w390:refnum<vi>[])
            }
            frame Default {
            }
          }
        }
        n201 = Greater Or Equal?(x=w373, y=3) -> (x >= y?=w371:bool)
        n202 = case shown="True" w371 {
          tunnel: w370 -> [w380 _]
          tunnel: [w380 _] -> w369
          frame False {
          }
          frame True {
            n203 = One Button Dialog(message="Cannot edit more than three\nremote files at the same time.") -> ()  [unwired: 1 in, 1 out]
          }
        }
      }
      frame "remote file" {
        n204 = vi-ref "re_Edit Remote File.vi"() -> ("vi reference"=w407:refnum<vi>)
        n205 = property class="VI Interface Type 3"(reference=w407) -> (error out=w400:errorcluster, "VI Name"=w406:string)  [unwired: 1 in, 1 out]
        n206 = Open VI Reference(vi path=w406, options=8, error in (no error)=w400) -> (vi reference=w402:refnum<vi>, error out=w401:errorcluster)  [unwired: 3 in]
        n207 = invoke class="VI" method="Run VI"(reference=w402, error in=w401, "Wait until done"=FALSE, "Auto Dispose Ref"=TRUE) -> (reference out=w398:refnum<vi>, error out=w399:errorcluster)  [unwired: 1 in, 3 out]
        n208 = case shown="Error" w399 {
          selector: w399 -> [_ w416]
          tunnel: w398 -> [w413 w414]
          tunnel: [w412 w415] -> w397
          tunnel: w396 -> [w411 w415]
          frame No Error {
            n209 = Build Array (concatenate)(w413, w411) -> (w412:refnum<vi>[])
          }
          frame Error {
            n210 = Close Reference(reference=w414) -> ()  [unwired: 1 in, 1 out]
            n211 = call "Library Log Error to Window.vi"("error in (no error)"=w416) -> ()  [unwired: 13 in, 2 out]
          }
        }
      }
      frame "connect" {
        n212 = local read "observer digest"() -> (w418:string)
        n213 = local read "machine name"() -> (w419:string)
        n214 = local read "port number"() -> (w420:u32)
        n215 = call "obj_ClientSrv Connection State.vi"("method (get state)"=t_ClientSrv_Connection_State_Methods."connect" ("method"), "machine{connect}/VI{get state} name (local/no path resolution)"=w419, "port number in (3363)"=w420, "observer digest"=w418) -> ("error out"=w421:errorcluster)  [unwired: 4 in, 7 out]
        n216 = case shown="No Error" w421 {
          selector: w421 -> [_ w428]
          tunnel: [w426 w427] -> w424
          frame No Error {
            w426 = T4[] [enum."open refs", enum."update presets", enum."update name", enum."update ablement", enum."start session", enum."run consoles"] items=["empty queue", "poll list selection", "browse editor", "set editor", "no editors?", "<3 editors?", "remote file", "connect", "stop session", "server stop", "server reboot", "disconnect", "open refs", "update presets", "update name", "update ablement", "update sizes", "start session", "run consoles", "initialize", "init title", "init disconnect", "init patience", "init persist", "init paths", "init list", "init sort", "init done", "cleanup", "stop"] ("Array Constant")
          }
          frame Error {
            w427 = T4[] [enum."update ablement"] items=["empty queue", "poll list selection", "browse editor", "set editor", "no editors?", "<3 editors?", "remote file", "connect", "stop session", "server stop", "server reboot", "disconnect", "open refs", "update presets", "update name", "update ablement", "update sizes", "start session", "run consoles", "initialize", "init title", "init disconnect", "init patience", "init persist", "init paths", "init list", "init sort", "init done", "cleanup", "stop"] ("Array Constant")
            n217 = call "Library Log Error to Window.vi"("error in (no error)"=w428) -> ()  [unwired: 13 in, 2 out]
          }
        }
      }
      frame "stop session" {
        n218 = flat-sequence {
          frame #0 {
            n219 = call <vilib>:"Set Busy.vi"() -> ()  [unwired: 10 in, 2 out]
          }
          frame #1 {
            n220 = call "obj_Library Session.vi"("method"=t_Library_Session_Methods."stop session") -> ("error out"=w433:errorcluster)  [unwired: 11 in, 3 out]
            n221 = while "wait for running VI's to clean up, timeout in 5s" {
              tunnel: w433 -> [_]
              i -> [w439]
              stop <- w435 stop-if-true
              n222 = call "obj_Library Session.vi"("method"=t_Library_Session_Methods."list empty?") -> ("cleanup/empty?"=w440:bool)  [unwired: 11 in, 3 out]
              n223 = Greater Or Equal?(x=w439, y=50) -> (x >= y?=w437:bool)
              n224 = Or(x=w440, y=w437) -> (x .or. y?=w436:bool)
              n225 = case shown="False" w436 {
                selector: w436 -> [w443 w444]
                tunnel: [w443 w444] -> w435
                frame False {
                  n226 = Wait (ms)(milliseconds to wait=u32 100) -> ()  [unwired: 1 out]
                }
                frame True {
                }
              }
            }
          }
          frame #2 {
            n227 = call <vilib>:"Unset Busy.vi"() -> ()  [unwired: 11 in, 1 out]
          }
        }
      }
      frame "server stop" {
        n228 = local read "runlevels"() -> (w448:T2)
        n229 = call "obj_ClientSrv Client Access State.vi"("access level (observer)"=t_ClientSrv_Access_Levels."operator") -> ("certificate"=w453:string, "error out"=w452:errorcluster)  [unwired: 13 in]
        n230 = call-by-ref "?"(reference=w448, error in=w452, "method"=t_ClientSrv_Server_Runlevels_Methods."change", "certificate"=w453, "runlevel/bootmode"="stop" ("runlevel")) -> (error out=w451:errorcluster, 15:"error out"=w450:errorcluster)  [unwired: 10 in, 3 out]
        n231 = call "Library Remote Call Error Merger.vi"("call by reference node error"=w451, "called VI error (no error)"=w450) -> ("error out"=w447:errorcluster)  [unwired: 13 in]
        n232 = call "Library Log Error to Window.vi"("error in (no error)"=w447) -> ()  [unwired: 13 in, 2 out]
      }
      frame "server reboot" {
        n233 = local read "runlevels"() -> (w461:T2)
        n234 = local read "rebootmode"() -> (w463:string)
        n235 = call "obj_ClientSrv Client Access State.vi"("access level (observer)"=t_ClientSrv_Access_Levels."operator") -> ("certificate"=w464:string, "error out"=w473:errorcluster)  [unwired: 13 in]
        n236 = call-by-ref "?"(reference=w461, error in=w473, "method"=t_ClientSrv_Server_Runlevels_Methods."set bootmode", "certificate"=w464, "runlevel/bootmode"=w463) -> (reference out=w459:T2, error out=w472:errorcluster, 15:"error out"=w471:errorcluster)  [unwired: 10 in, 2 out]
        n237 = call "Library Remote Call Error Merger.vi"("call by reference node error"=w472, "called VI error (no error)"=w471) -> ("error out"=w466:errorcluster)  [unwired: 13 in]
        n238 = call-by-ref "?"(reference=w459, error in=w466, "method"=t_ClientSrv_Server_Runlevels_Methods."change", "certificate"=w464, "runlevel/bootmode"="reboot" ("runlevel")) -> (error out=w468:errorcluster, 15:"error out"=w469:errorcluster)  [unwired: 10 in, 3 out]
        n239 = call "Library Remote Call Error Merger.vi"("call by reference node error"=w468, "called VI error (no error)"=w469) -> ("error out"=w465:errorcluster)  [unwired: 13 in]
        n240 = call "Library Log Error to Window.vi"("error in (no error)"=w465) -> ()  [unwired: 13 in, 2 out]
      }
      frame "disconnect" {
        n241 = call "obj_ClientSrv Connection State.vi"() -> ("connected?"=w478:bool)  [unwired: 8 in, 7 out]
        n242 = case "connected?" shown="True" w478 {
          frame False {
          }
          frame True {
            n243 = flat-sequence {
              frame #0 {
                n244 = local read "runlevels"() -> (w483:T2)
                n245 = local read "info"() -> (w482:T1)
                n246 = Close Reference(reference=w483) -> ()  [unwired: 1 in, 1 out]
                n247 = Close Reference(reference=w482) -> ()  [unwired: 1 in, 1 out]
              }
              frame #1 {
                n248 = local write "runlevels"(T2 refnum ("runlevels")) -> ()
                n249 = local write "info"(T1 refnum ("info")) -> ()
              }
              frame #2 {
                n250 = call "obj_ClientSrv Client Access State.vi"("method (ensure)"=t_ClientSrv_Client_Access_State_Methods."release") -> ()  [unwired: 13 in, 2 out]
              }
              frame #3 {
                n251 = local write "server"("") -> ()
                n252 = call "obj_ClientSrv Connection State.vi"("method (get state)"=t_ClientSrv_Connection_State_Methods."disconnect" ("method")) -> ()  [unwired: 7 in, 8 out]
              }
            }
          }
        }
      }
      frame "open refs" {
        n253 = call "obj_ClientSrv Connection State.vi"("machine{connect}/VI{get state} name (local/no path resolution)"="ClientSrv Server Runlevels_srv.vi") -> ("server app ref"=w497:refnum<vi>, "resolved server path"=w498:path, "error out"=w499:errorcluster)  [unwired: 7 in, 5 out]
        n254 = local read "runlevels"() -> (w496:T2)
        n255 = stacked-sequence {
          tunnel: [w535] -> w495
          tunnel: [w534] -> w500
          tunnel: w499 -> [w533]
          tunnel: w497 -> [w532]
          tunnel: w498 -> [w531]
          tunnel: w496 -> [w530]
          frame #0 {
            # "avoid LV8 complaints"
            n256 = Path to Array of Strings(0:w531) -> (2:w536:string[])  [unwired: 1 out]
            n257 = Array Size(array=w536) -> (size(s)=w537:i32)
            n258 = case shown="1" w537 {
              tunnel: w531 -> [w544 w550]
              tunnel: w532 -> [w542 w549]
              tunnel: [w540 w545] -> w535
              tunnel: [w538 w548] -> w534
              tunnel: w530 -> [w539 w547]
              tunnel: w533 -> [w541 w546]
              frame 1 {
                n259 = Path To String(path=w544) -> (string=w543:string)
                n260 = Open VI Reference(type specifier VI Refnum (for type only)=w539, application reference (local)=w542, vi path=w543, error in (no error)=w541) -> (vi reference=w540:T2, error out=w538:errorcluster)  [unwired: 2 in]
              }
              frame Default {
                n261 = Open VI Reference(type specifier VI Refnum (for type only)=w547, application reference (local)=w549, vi path=w550, error in (no error)=w546) -> (vi reference=w545:T2, error out=w548:errorcluster)  [unwired: 2 in]
              }
            }
          }
        }
        "runlevels" <- w495
        n262 = call "Library Open VI Ref Error Clarifier.vi"("VI path"=w498, "called VI error (no error)"=w500) -> ("error out"=w503:errorcluster)  [unwired: 13 in]
        n263 = call "obj_ClientSrv Connection State.vi"("machine{connect}/VI{get state} name (local/no path resolution)"="LuaVIEW Info_srv.vi", "error in (no error)"=w503) -> ("server app ref"=w492:refnum<vi>, "resolved server path"=w491:path, "error out"=w493:errorcluster)  [unwired: 6 in, 5 out]
        n264 = local read "info"() -> (w490:T1)
        n265 = stacked-sequence {
          tunnel: [w514] -> w489
          tunnel: [w513] -> w494
          tunnel: w493 -> [w512]
          tunnel: w492 -> [w511]
          tunnel: w491 -> [w510]
          tunnel: w490 -> [w509]
          frame #0 {
            # "avoid LV8 complaints"
            n266 = Path to Array of Strings(0:w510) -> (2:w515:string[])  [unwired: 1 out]
            n267 = Array Size(array=w515) -> (size(s)=w516:i32)
            n268 = case shown="1" w516 {
              tunnel: w510 -> [w523 w529]
              tunnel: w511 -> [w521 w528]
              tunnel: [w519 w524] -> w514
              tunnel: [w517 w527] -> w513
              tunnel: w509 -> [w518 w526]
              tunnel: w512 -> [w520 w525]
              frame 1 {
                n269 = Path To String(path=w523) -> (string=w522:string)
                n270 = Open VI Reference(type specifier VI Refnum (for type only)=w518, application reference (local)=w521, vi path=w522, error in (no error)=w520) -> (vi reference=w519:T1, error out=w517:errorcluster)  [unwired: 2 in]
              }
              frame Default {
                n271 = Open VI Reference(type specifier VI Refnum (for type only)=w526, application reference (local)=w528, vi path=w529, error in (no error)=w525) -> (vi reference=w524:T1, error out=w527:errorcluster)  [unwired: 2 in]
              }
            }
          }
        }
        "info" <- w489
        n272 = call "Library Open VI Ref Error Clarifier.vi"("VI path"=w491, "called VI error (no error)"=w494) -> ("error out"=w502:errorcluster)  [unwired: 13 in]
        n273 = call "Library Log Error to Window.vi"("error in (no error)"=w502) -> ()  [unwired: 13 in, 2 out]
      }
      frame "update presets" {
        # "avoid LV7 bug"
        n274 = local read "machine name"() -> (w562:string)
        n275 = local read "port number"() -> (w561:u32)
        n276 = call "obj_ClientSrv Connection State.vi"() -> ("server"=w569:string)  [unwired: 8 in, 7 out]
        n277 = local read "presets"() -> (w555:T3)
        n278 = Reshape Array(w555, 0 ("dimension size")) -> (w556:T3)
        n279 = Index Array(array=w555, index=-1) -> (element=w566:T13)
        n280 = local read "remember"() -> (w557:bool)
        n281 = for "delete colliding entries" {
          tunnel: w555 -> [w572] mode=indexing
          shift-right: [w587] -> w564
          shift-left: w556 -> [w586]
          tunnel: w569 -> [w584]
          tunnel: w562 -> [w582]
          tunnel: w561 -> [w578]
          n282 = To Lower Case(string=w582) -> (all lower case string=w580:string)
          n283 = Unbundle By Name(w572) -> ("server"=w585:string, "machine"=w583:string, "port"=w579:u32)
          n284 = To Lower Case(string=w583) -> (all lower case string=w581:string)
          n285 = Equal?(x=w584, y=w585) -> (x = y?=w575:bool)
          n286 = Equal?(x=w580, y=w581) -> (x = y?=w576:bool)
          n287 = Equal?(x=w578, y=w579) -> (x = y?=w577:bool)
          n288 = And(x=w576, y=w577) -> (x .and. y?=w574:bool)
          n289 = Or(x=w575, y=w574) -> (x .or. y?=w573:bool)
          n290 = case shown="False" w573 {
            tunnel: [w589 w591] -> w587
            tunnel: w586 -> [w590 w591]
            tunnel: w572 -> [w588 _]
            frame False {
              n291 = Build Array (concatenate)(w590, w588) -> (w589:T3)
            }
            frame True {
            }
          }
        }
        n292 = local read "observer digest"() -> (w558:string)
        n293 = Select(t=w558, s=w557, f="") -> (s? t:f=w560:string)
        n294 = Bundle By Name(cluster=w566, "server"=w569, "machine"=w562, "port"=w561, "digest"=w560, "remember"=w557) -> (w565:T13)
        n295 = Build Array (concatenate)(w565, w564) -> (w553:T3)
        n296 = Sort 1D Array(array=w553) -> (sorted array=w552:T3)
        n297 = Sort 1D Array(array=w552) -> (sorted array=w563:T3)
        n298 = local write "presets"(w563) -> ()
      }
      frame "update name" {
        n299 = local read "runlevels"() -> (w597:T2)
        n300 = call "obj_ClientSrv Client Access State.vi"() -> ("certificate"=w601:string, "error out"=w600:errorcluster)  [unwired: 14 in]
        n301 = call-by-ref "?"(reference=w597, error in=w600, "method"=t_ClientSrv_Server_Runlevels_Methods."get modes", "certificate"=w601) -> (error out=w599:errorcluster, "current"=w593:string, 15:"error out"=w598:errorcluster)  [unwired: 11 in, 2 out]
        n302 = call "obj_ClientSrv Connection State.vi"() -> ("server"=w595:string)  [unwired: 8 in, 7 out]
        n303 = call "Library Remote Call Error Merger.vi"("call by reference node error"=w599, "called VI error (no error)"=w598) -> ("error out"=w596:errorcluster)  [unwired: 13 in]
        n304 = case shown="No Error" w596 {
          selector: w596 -> [_ w617]
          tunnel: w595 -> [w609 w616]
          tunnel: [w608 w616] -> w594
          tunnel: w593 -> [w606 _]
          frame No Error {
            n305 = Empty String/Path?(string/path=w606) -> (empty?=w607:bool)
            n306 = case shown="False" w607 {
              tunnel: w609 -> [w614 w615]
              tunnel: [w613 w615] -> w608
              tunnel: w606 -> [w612 _]
              frame False {
                n307 = Concatenate Strings(w614, " (" ("string"), w612, ")" ("string")) -> (w613:string)
              }
              frame True {
              }
            }
          }
          frame Error {
            n308 = call "Library Log Error to Window.vi"("error in (no error)"=w617) -> ()  [unwired: 13 in, 2 out]
          }
        }
        "server" <- w594
      }
      frame "update ablement" {
        w629 = "Remove Preset" ("menu tag")
        w643 = u8 2 items=["enabled", "disabled", "grayed"] ("disabled state")
        w625 = "Server Presets" ("menu tag")
        w644 = u8 0 items=["enabled", "disabled", "grayed"] ("disabled state")
        n309 = for {
          tunnel: "presets" -> [w659] mode=indexing
          tunnel: [w658] -> w634 mode=indexing
          tunnel: [w656] -> w624 mode=indexing
          tunnel: [w653] -> w639 mode=indexing
          i -> [w654]
          n310 = Unbundle By Name(w659) -> ("server"=w658:string)
          n311 = Format Into String(format string="Preset%d", w654) -> (resulting string=w656:string)  [unwired: 2 in, 1 out]
          n312 = Format Into String(format string="Remove%d", w654) -> (resulting string=w653:string)  [unwired: 2 in, 1 out]
        }
        n313 = Current VI's Menubar() -> (w641:refnum<k9>)
        n314 = Array Size(array="presets") -> (size(s)=w623:i32)
        n315 = Greater Than 0?(x=w623) -> (x > 0?=w620:bool)
        n316 = Delete Menu Items(8:w625, 9:w641) -> (3:w635:refnum<k9>)  [unwired: 2 in, 1 out]
        n317 = call "obj_ClientSrv Connection State.vi"() -> ("connected?"=w619:bool)  [unwired: 8 in, 7 out]
        n318 = Insert Menu Items(5:w625, 7:w624, 8:w634, 9:w635) -> (3:w627:refnum<k9>)  [unwired: 2 in, 2 out]
        n319 = Not(x=w619) -> (.not. x?=w645:bool)
        n320 = Compound Arithmetic op=AND(invert w619, w620) -> (w621:bool)
        n321 = property class="VI"("Front Panel Window:Closeable"=w645) -> ()  [unwired: 2 in, 2 out]
        n322 = Set Menu Item Info(7:w625, 9:w621, 11:w627) -> (3:w626:refnum<k9>)  [unwired: 4 in, 1 out]
        n323 = Delete Menu Items(8:w629, 9:w626) -> (3:w640:refnum<k9>)  [unwired: 2 in, 1 out]
        n324 = Insert Menu Items(5:w629, 7:w639, 8:w634, 9:w640) -> (3:w630:refnum<k9>)  [unwired: 2 in, 2 out]
        n325 = Set Menu Item Info(7:w629, 9:w620, 11:w630) -> (3:w628:refnum<k9>)  [unwired: 4 in, 1 out]
        n326 = Not(x=w619) -> (.not. x?=w637:bool)
        n327 = Set Menu Item Info(7:"Connect" ("item tag"), 9:w637, 11:w628) -> (3:w632:refnum<k9>)  [unwired: 4 in, 1 out]
        n328 = for {
          tunnel: w619 -> [w652]
          shift-right: [w650] -> w631
          shift-left: w632 -> [w651]
          tunnel: string[] ["Disconnect", "Release Access", "Runlevels", "Show Server Info", "Show Server Errors", "Show Server Warnings", "Remote File"] -> [w649] mode=indexing
          n329 = Set Menu Item Info(7:w649, 9:w652, 11:w651) -> (3:w650:refnum<k9>)  [unwired: 4 in, 1 out]
        }
        n330 = Select(t=w644, s=w619, f=w643) -> (s? t:f=w642:u8)
        n331 = property on="list" class="LstBox (strict)"("Disabled"=w642) -> ()  [unwired: 2 in, 2 out]
        n332 = Enable Menu Tracking(3:TRUE ("enable (T)"), 4:w631) -> ()  [unwired: 1 in, 2 out]
      }
      frame "update sizes" {
        n333 = property on="list" class="LstBox (strict)"() -> ("Position:Left"=w661:i32, "Bounds:Width"=w664:u32)  [unwired: 2 in, 2 out]
        n334 = property on="server" class="Str"() -> ("Bounds:Width"=w666:u32, "Text.Size:Width"=w665:u32)  [unwired: 2 in, 2 out]
        n335 = Subtract(x=w666, y=w665) -> (x-y=w663:u32)
        n336 = Subtract(x=w664, y=w663) -> (x-y=w662:u32)
        n337 = property on="server" class="Str"("Position:Left"=w661, "Text.Size:Width"=w662) -> ()  [unwired: 2 in, 2 out]
      }
      frame "start session" {
        n338 = call "obj_Library Session.vi"("method"=t_Library_Session_Methods."start session") -> ()  [unwired: 11 in, 4 out]
      }
      frame "run consoles" {
        # "By running the console windows of the errors and warnings\ntask in the background, the windows will pop-up when a\nserver-side warning or error occurs."
        n339 = Flatten To String(anything=T8 {"open on start"=FALSE, "stop on close"=FALSE, "hide initial"=TRUE, "timeout"=0} ("task console ancillary")) -> (data string=w676:string)  [unwired: 3 in, 2 out]
        n340 = call "Library Resolve VI Path.vi"("VI name"="ui_LuaVIEW Task Console.vit", "sub path of toolkit (none)"=path "dynamic" ("subdirectory of tree (none)")) -> ("VI path"=w677:path)  [unwired: 13 in]
        n341 = call "obj_Library Session.vi"("method"=t_Library_Session_Methods."run", "path"=w677, "argument in (none)"="warnings", "ancillary in (none)"=w676) -> ("error out"=w683:errorcluster)  [unwired: 8 in, 3 out]
        n342 = call "obj_Library Session.vi"("method"=t_Library_Session_Methods."run", "path"=w677, "argument in (none)"="errors", "ancillary in (none)"=w676) -> ("error out"=w679:errorcluster)  [unwired: 8 in, 3 out]
        n343 = call "Library Log Error to Window.vi"("error in (no error)"=w683) -> ()  [unwired: 13 in, 2 out]
        n344 = call "Library Log Error to Window.vi"("error in (no error)"=w679) -> ()  [unwired: 13 in, 2 out]
      }
      frame "initialize" {
        n345 = while "rebuild init list on first run or after load or recompile" {
          shift-left: _ -> [w696]
          shift-right: [w695] -> w693
          stop <- FALSE continue-if-true
          n346 = Array Size(array=w696) -> (size(s)=w697:i32)
          n347 = case shown="0" w697 {
            tunnel: [w698 w718] -> w695
            tunnel: w696 -> [w699 w718]
            frame 0 {
              n348 = while {
                shift-left: w699 -> [w708]
                shift-right: [w706] -> w698
                shift-left: _ -> [w710]
                shift-right: [w705] -> _
                i -> [w713]
                stop <- w701 continue-if-true
                n349 = To Unsigned Word Integer(number=w713) -> (unsigned 16bit integer=w711:u16)
                n350 = Type Cast(type=t_ClientSrv_Client_Main_States."initialize" ("states"), x=w711) -> (*(type *) &x=w707:T4)
                n351 = Format Into String(format string="%s" ("Format String"), w707) -> (resulting string=w705:string)  [unwired: 2 in, 1 out]
                n352 = Not Equal?(x=w705, y=w710) -> (x != y?=w701:bool)
                n353 = Match Pattern(string=w705, regular expression="^init ") -> (offset past match=w703:i32)  [unwired: 1 in, 3 out]
                n354 = Greater Or Equal To 0?(x=w703) -> (x >= 0?=w702:bool)
                n355 = And(x=w702, y=w701) -> (x .and. y?=w700:bool)
                n356 = case shown="True" w700 {
                  tunnel: w708 -> [w714 w717]
                  tunnel: w707 -> [_ w716]
                  tunnel: [w714 w715] -> w706
                  frame False {
                  }
                  frame True {
                    n357 = Build Array (concatenate)(w717, w716) -> (w715:T4[])
                  }
                }
              }
            }
            frame Default {
            }
          }
        }
      }
      frame "init title" {
        n358 = property class="VI"("Front Panel Window:Title"="Client") -> (reference out=w720:refnum<vi>)  [unwired: 2 in, 1 out]
        n359 = global write "glb_ClientSrv Globals.vi" "client VI ref"(w720) -> ()
      }
      frame "init disconnect" {
        # "Drop any test connection that could still be active."
        n360 = call "obj_ClientSrv Connection State.vi"("method (get state)"=t_ClientSrv_Connection_State_Methods."disconnect" ("method")) -> ()  [unwired: 7 in, 8 out]
      }
      frame "init patience" {
        w734 = u8 2 items=["enabled", "disabled", "grayed"] ("disabled state")
        n361 = Current VI's Menubar() -> (w733:refnum<k9>)
        n362 = property on="list" class="LstBox (strict)"("Disabled"=w734) -> ()  [unwired: 2 in, 2 out]
        n363 = local write "server"("Initializing...") -> ()
        n364 = Enable Menu Tracking(3:FALSE ("enable (T)"), 4:w733) -> ()  [unwired: 1 in, 2 out]
      }
      frame "init persist" {
        n365 = call "Libary Persist Position and Controls.vi"("action"=enum16{"save", "load"}."load", "filename (<window title hash>.dat)"=w742) -> ()  [unwired: 12 in, 2 out]
        n366 = Build Array (concatenate)(t_ClientSrv_Client_Main_States."update sizes" ("states"), w741) -> (w740:T4[])
      }
      frame "init paths" {
        w751 = T4[] [enum."cleanup"] items=["empty queue", "poll list selection", "browse editor", "set editor", "no editors?", "<3 editors?", "remote file", "connect", "stop session", "server stop", "server reboot", "disconnect", "open refs", "update presets", "update name", "update ablement", "update sizes", "start session", "run consoles", "initialize", "init title", "init disconnect", "init patience", "init persist", "init paths", "init list", "init sort", "init done", "cleanup", "stop"] ("Array Constant")
        n367 = property class="App"() -> ("App.Kind"=w746:T11)  [unwired: 2 in, 2 out]
        n368 = case shown="\"Run Time System\"" w746 {
          tunnel: [path[] [path "tui_ClientSrv Remote File Manager.vi", path "tui_DataLog Live Tag Chart.vit", path "tui_DataLog Live Tag Table.vit", path "tui_DataLog Log Book.vit", path "tui_DataLog Log Graph.vit", path "tui_DataLog Log Table.vi", path "tui_DataLog Tag Manager.vi", path "tui_Datalog Tag Subset Editor.vi", path "tui_LuaVIEW Function Manager.vi", path "tui_LuaVIEW Task Manager.vi"] ("Array") w757] -> w750
          tunnel: [_ w755] -> w748
          frame "Run Time System" {
            # "This hack gets around the problem of LabVIEW being unable to list the VI's\ninside the executable as of LabVIEW 8.2"
          }
          frame Default {
            n369 = flat-sequence {
              tunnel: [w762] -> w757
              tunnel: [w759] -> w758
              tunnel: [w764] -> w756
              tunnel: w758 -> [w764]
              frame #0 {
                n370 = call <vilib>:"Set Busy.vi"() -> ()  [unwired: 10 in, 2 out]
              }
              frame #1 {
                n371 = call "Library Toolkit Path.vi"() -> ("absolute toolkit path"=w760:path)  [unwired: 15 in]
                n372 = call "Library Recursively List Files.vi"("root directory"=w760, "enter llbs? (no)"=TRUE, "pattern (none)"="tui_*.*") -> ("file list"=w762:path[], "error out"=w759:errorcluster)  [unwired: 10 in, 1 out]
              }
              frame #2 {
                n373 = call <vilib>:"Unset Busy.vi"() -> ()  [unwired: 11 in, 1 out]
              }
            }
            n374 = call "Library Log Error to Window.vi"("error in (no error)"=w756) -> ("dup error"=w755:errorcluster)  [unwired: 13 in, 1 out]
          }
        }
        n375 = Select(t=w751, s=w748, f=w752) -> (s? t:f=w753:T4[])
      }
      frame "init list" {
        w769 = T4[] [enum."cleanup"] items=["empty queue", "poll list selection", "browse editor", "set editor", "no editors?", "<3 editors?", "remote file", "connect", "stop session", "server stop", "server reboot", "disconnect", "open refs", "update presets", "update name", "update ablement", "update sizes", "start session", "run consoles", "initialize", "init title", "init disconnect", "init patience", "init persist", "init paths", "init list", "init sort", "init done", "cleanup", "stop"] ("Array Constant")
        n376 = stacked-sequence {
          tunnel: [_ w776 _] -> w768
          tunnel: w767 -> [_ w775 _]
          tunnel: [_ w773 _] -> w766
          frame #0 {
            n377 = call <vilib>:"Set Busy.vi"() -> ()  [unwired: 10 in, 2 out]
          }
          frame #1 {
            n378 = for {
              shift-right: [w797] -> w776
              shift-left: errorcluster {"status"=FALSE, "code"=0, "source"=""} ("error IO") -> [w796]
              tunnel: w775 -> [w794] mode=indexing
              shift-right: [w784] -> _
              shift-left: string[] [] -> [w795]
              shift-right: [w787] -> w773
              shift-left: refnum<vi>[] [] -> [w788]
              w778 = FALSE  # preload if not a template?
              # "preloading improves performance after\ninitialisation, but eats up memory."
              # "When you enable preloading below, make\nsure all GUI VIs clean up their controls and\nindicators on exit because the front panel\nwill remain loaded. Also note that control\npositioning errors because of window\nresizing hysterisis will accumulate."
              # "strip \"tui_<toolkit>\" prefix and \".vi\" or \".vit\" postfix"
              n379 = Strip Path(path=w794) -> (name=w793:string)  [unwired: 1 out]
              n380 = Match Pattern(string=w793, regular expression="\\s") -> (after substring=w783:string)  [unwired: 1 in, 3 out]
              n381 = Match Pattern(string=w783, regular expression=".[vV][iI][tT]?$") -> (before substring=w790:string, match substring=w789:string)  [unwired: 1 in, 2 out]
              n382 = String Length(string=w789) -> (length=w782:i32)
              n383 = Not Equal?(x=w782, y=4) -> (x != y?=w780:bool)
              n384 = And(x=w778, y=w780) -> (x .and. y?=w779:bool)
              n385 = case "preload?" shown="False" w779 {
                tunnel: [w798 w810] -> w797
                tunnel: w796 -> [w798 w809]
                tunnel: [w800 w808] -> w786
                tunnel: w795 -> [w800 w807]
                tunnel: w794 -> [_ w806]
                tunnel: w790 -> [w801 w805]
                tunnel: w788 -> [w799 w804]
                tunnel: [w799 w803] -> w787
                tunnel: [w801 w802] -> w785
                frame False {
                }
                frame True {
                  n386 = case shown="No Error" w809 {
                    selector: w809 -> [w821 w842]
                    tunnel: [w819 w842] -> w810
                    tunnel: w806 -> [w811 _]
                    tunnel: [w817 w841] -> w808
                    tunnel: w807 -> [w816 w841]
                    tunnel: w805 -> [w815 w840]
                    tunnel: [w814 w840] -> w802
                    tunnel: w804 -> [w813 w839]
                    tunnel: [w812 w839] -> w803
                    frame No Error {
                      n387 = Open VI Reference(vi path=w811, error in (no error)=w821) -> (vi reference=w818:refnum<vi>, error out=w820:errorcluster)  [unwired: 4 in]
                      n388 = case shown="No Error" w820 {
                        selector: w820 -> [w832 w835]
                        tunnel: [w830 w834] -> w819
                        tunnel: w818 -> [w829 _]
                        tunnel: [w824 w838] -> w817
                        tunnel: w816 -> [w824 w838]
                        tunnel: w815 -> [w828 w837]
                        tunnel: [w825 w837] -> w814
                        tunnel: w813 -> [w823 w836]
                        tunnel: [w822 w836] -> w812
                        tunnel: w811 -> [_ w833]
                        frame No Error {
                          n389 = property class="VI"(reference=w829, error in=w832) -> (reference out=w831:refnum<vi>, error out=w830:errorcluster, "Front Panel Window:Title"=w826:string, "Front Panel Window:Custom Title"=w827:bool)
                          n390 = Build Array (concatenate)(w823, w831) -> (w822:refnum<vi>[])
                          n391 = Select(t=w826, s=w827, f=w828) -> (s? t:f=w825:string)
                        }
                        frame Error {
                          n392 = call "Library Open VI Ref Error Clarifier.vi"("VI path"=w833, "called VI error (no error)"=w835) -> ("error out"=w834:errorcluster)  [unwired: 13 in]
                        }
                      }
                    }
                    frame Error {
                    }
                  }
                }
              }
              n393 = Build Array (concatenate)(w786, w785) -> (w784:string[])
              n394 = property on="list" class="LstBox (strict)"("Item Names"=w784) -> ()  [unwired: 2 in, 2 out]
            }
          }
          frame #2 {
            n395 = call <vilib>:"Unset Busy.vi"() -> ()  [unwired: 11 in, 1 out]
          }
        }
        n396 = call "Library Log Error to Window.vi"("error in (no error)"=w768) -> ()  [unwired: 13 in, 2 out]
        n397 = Select(t=w769, s=w768, f=w770) -> (s? t:f=w771:T4[])
      }
      frame "init sort" {
        # "avoid LV7 bug"
        n398 = property on="list" class="LstBox (strict)"() -> ("Item Names"=w851:string[])  [unwired: 2 in, 2 out]
        n399 = for {
          tunnel: w851 -> [w858] mode=indexing
          tunnel: w848 -> [w860]
          tunnel: [w856] -> w850 mode=indexing
          i -> [w859]
          n400 = Index Array(array=w860, index=w859) -> (element=w857:path)
          n401 = Bundle(w858, w857) -> (w856:cluster{string, path})  [unwired: 1 in]
        }
        n402 = Sort 1D Array(array=w850) -> (sorted array=w845:cluster{string, path}[])
        n403 = Sort 1D Array(array=w845) -> (sorted array=w844:cluster{string, path}[])
        n404 = for {
          tunnel: w844 -> [w855] mode=indexing
          tunnel: [w854] -> w847 mode=indexing
          tunnel: [w853] -> w849 mode=indexing
          n405 = Unbundle(w855) -> (w853:string, w854:path)
        }
        n406 = property on="list" class="LstBox (strict)"("Item Names"=w849) -> ()  [unwired: 2 in, 2 out]
      }
      frame "init done" {
        n407 = local write "server"("") -> ()
        n408 = Build Array (concatenate)(t_ClientSrv_Client_Main_States."update ablement" ("states"), w866) -> (w865:T4[])
      }
      frame "cleanup" {
        w872 = u8 2 items=["enabled", "disabled", "grayed"] ("disabled state")
        w882 = T4[] [enum."stop"] items=["empty queue", "poll list selection", "browse editor", "set editor", "no editors?", "<3 editors?", "remote file", "connect", "stop session", "server stop", "server reboot", "disconnect", "open refs", "update presets", "update name", "update ablement", "update sizes", "start session", "run consoles", "initialize", "init title", "init disconnect", "init patience", "init persist", "init paths", "init list", "init sort", "init done", "cleanup", "stop"] ("Array Constant")
        n409 = call "Libary Persist Position and Controls.vi"("action"=enum16{"save", "load"}."save", "filename (<window title hash>.dat)"=w871) -> ()  [unwired: 12 in, 2 out]
        n410 = for "close any open panels and unload preloaded VIs" {
          tunnel: w876 -> [w883] mode=indexing
          n411 = Not A Number/Path/Refnum?(number/path/refnum=w883) -> (NaN/Path/Refnum?=w884:bool)
          n412 = case shown="False" w884 {
            tunnel: w883 -> [w886 _]
            frame False {
              n413 = invoke class="VI" method="FP.Close"(reference=w886) -> (reference out=w885:refnum<vi>)  [unwired: 2 in, 2 out]
              n414 = Close Reference(reference=w885) -> ()  [unwired: 1 in, 1 out]
            }
            frame True {
            }
          }
        }
        n415 = global write "glb_ClientSrv Globals.vi" "client VI ref"(refnum<vi> refnum ("client VI ref")) -> ()
        n416 = local write "server"("") -> ()
        n417 = property on="list" class="LstBox (strict)"("Disabled"=w872, "Item Names"=string[] [], "Value"=-1 ("list")) -> ()  [unwired: 2 in, 2 out]
        n418 = Reshape Array(w876, 0 ("dimension size")) -> (w875:refnum<vi>[])
        n419 = Reshape Array(w877, 0 ("dimension size")) -> (w878:path[])
      }
      frame "stop" {
        # "avoid warning"
        n420 = property class="App"() -> ("Application:Kind"=w891:T11)  [unwired: 2 in, 2 out]
        n421 = case shown="Default" w891 {
          tunnel: "list" -> [_ _]
          frame "Run Time System" {
            n422 = invoke class="VI" method="FP.Close"() -> ()  [unwired: 3 in, 3 out]
          }
          frame Default {
          }
        }
      }
    }
  }
